vi "UART Close.vi"(8 "error in (no error)":errorcluster) -> (0 "error out":errorcluster)   [LabVIEW 2015]
uses:
  Libraries/uart_library.dll
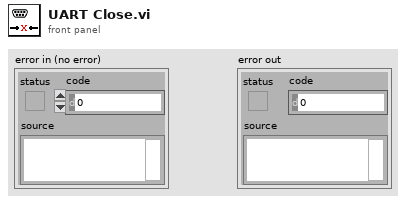
[diagram p1: front panel]
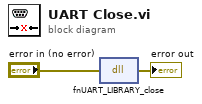
[diagram p0: block diagram]
diagram:
  n1 = dll-call lib="C:/Users/Labmember/Desktop/2psoftware - unstable/ScanningmiscroscopeDAQ/SubVis/Filter Wheel SubVI/Libraries/uart_library.dll" fn="fnUART_LIBRARY_close"(error in="error in (no error)") -> (error out=→"error out":errorcluster)  [unwired: 3 in, 1 out]
